vi "Get UDV Section from System Definition.vi"(8 "error in (no error)":errorcluster, 11 "System Definition Path":path) -> (0 "error out":errorcluster, 3 "NodeID":u64)   [LabVIEW 2019, in "Scan Engine EtherCAT System Tests.lvclass"]
uses:
  Scan Engine EtherCAT System Tests.lvclass
  NationalInstruments.VeriStand.SystemDefinitionAPI
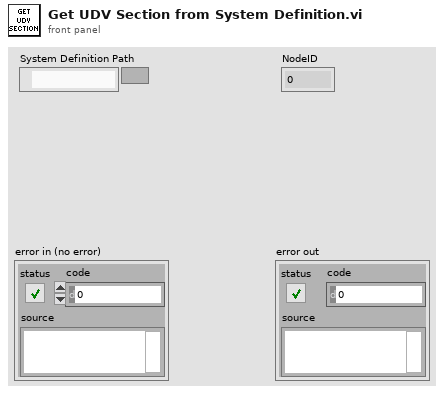
[diagram p1: front panel]
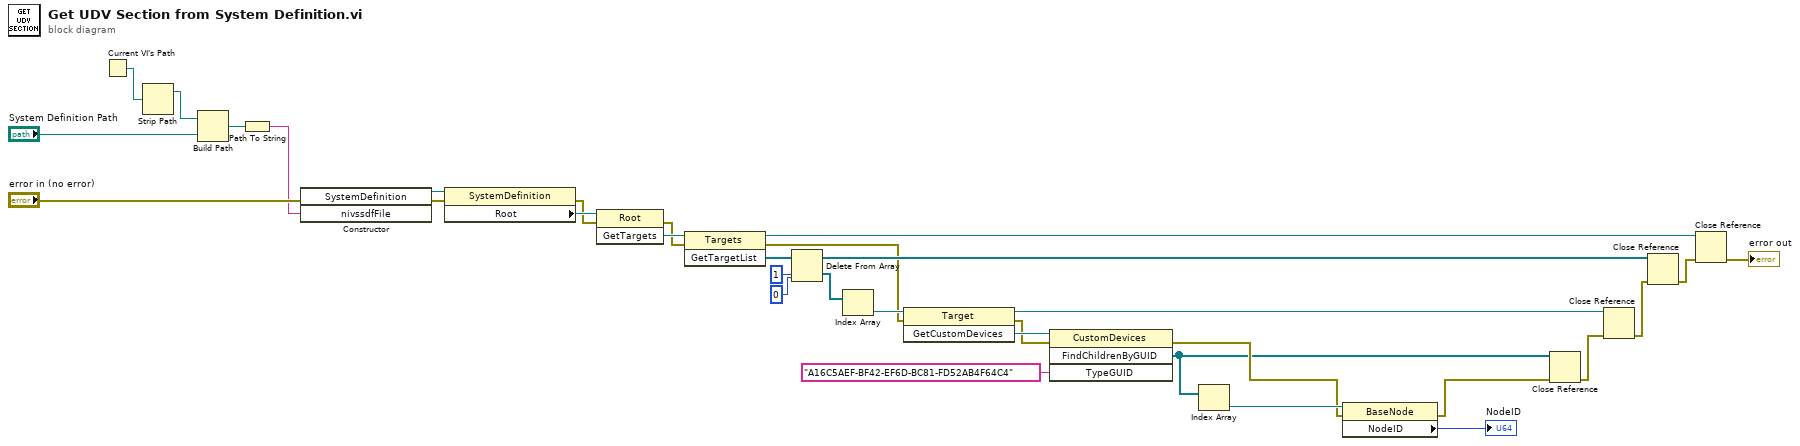
[diagram p0: block diagram]
diagram:
  n1 = Current VI's Path() -> (path=w11:path)
  n2 = Strip Path(path=w11) -> (stripped path=w10:path)  [unwired: 1 out]
  n3 = Build Path(base path=w10, name or relative path="System Definition Path") -> (appended path=w17:path)
  n4 = Path To String(path=w17) -> (string=w19:string)
  n5 = constructor class="SystemDefinition"(error in="error in (no error)", "nivssdfFile"=w19) -> (reference out=w22:refnum<k24>, error out=w21:errorcluster)  [unwired: 2 in, 2 out]
  n6 = property class="SystemDefinition"(reference=w22, error in=w21) -> (error out=w23:errorcluster, "Root"=w24:refnum<k24>)  [unwired: 1 out]
  n7 = invoke class="Root" method="GetTargets"(reference=w24, error in=w23) -> (error out=w25:errorcluster, "GetTargets"=w26:refnum<k24>)  [unwired: 1 in, 1 out]
  n8 = invoke class="Targets" method="GetTargetList"(reference=w26, error in=w25) -> (reference out=w32:refnum<k24>, error out=w9:errorcluster, "GetTargetList"=w27:refnum<k24>[])  [unwired: 1 in]
  n9 = Delete From Array(array=w27, length=1, index=0) -> (deleted portion=w33:refnum<k24>[], array with subset deleted=w30:refnum<k24>[])
  n10 = Index Array(array=w33) -> (element=w16:refnum<k24>)  [unwired: 1 in]
  n11 = invoke class="Target" method="GetCustomDevices"(reference=w16, error in=w9) -> (reference out=w7:refnum<k24>, error out=w8:errorcluster, "GetCustomDevices"=w15:refnum<k24>)  [unwired: 1 in]
  n12 = invoke class="CustomDevices" method="FindChildrenByGUID"(reference=w15, error in=w8, "TypeGUID"="A16C5AEF-BF42-EF6D-BC81-FD52AB4F64C4") -> (error out=w6:errorcluster, "FindChildrenByGUID"=w5:refnum<k24>[])  [unwired: 1 in, 2 out]
  n13 = Index Array(array=w5) -> (element=w13:refnum<k24>)  [unwired: 1 in]
  n14 = property class="BaseNode"(reference=w13, error in=w6) -> (error out=w4:errorcluster, "NodeID"=→"NodeID":u64)  [unwired: 1 out]
  n15 = Close Reference(reference=w5, error in (no error)=w4) -> (error out=w3:errorcluster)
  n16 = Close Reference(reference=w7, error in (no error)=w3) -> (error out=w2:errorcluster)
  n17 = Close Reference(reference=w30, error in (no error)=w2) -> (error out=w31:errorcluster)
  n18 = Close Reference(reference=w32, error in (no error)=w31) -> (error out=→"error out":errorcluster)
